vi "INIT.vi"(8 "error in (no error)":errorcluster, 11 "Emulate in":refnum<class "Emulate.lvclass">) -> (0 "error out":errorcluster, 3 "Emulate out":refnum<class "Emulate.lvclass">)   [LabVIEW 2020, in "Emulate.lvclass"]
uses:
  Emulate.lvclass
  C:/Dev/TRANCON/Classes/GeneralFunctionality/GeneralFunctionality.lvclass
  C:/Dev/TRANCON/Classes/Detector/Detector.lvclass
  GeneralFunctionality/GeneralFunctionality.lvclass/GeneralFunctionality.ctl
  Config/Config.lvclass
  Detector.lvclass
  Emulate.lvclass/Emulate.ctl
  GeneralFunctionality/GeneralFunctionality.lvclass
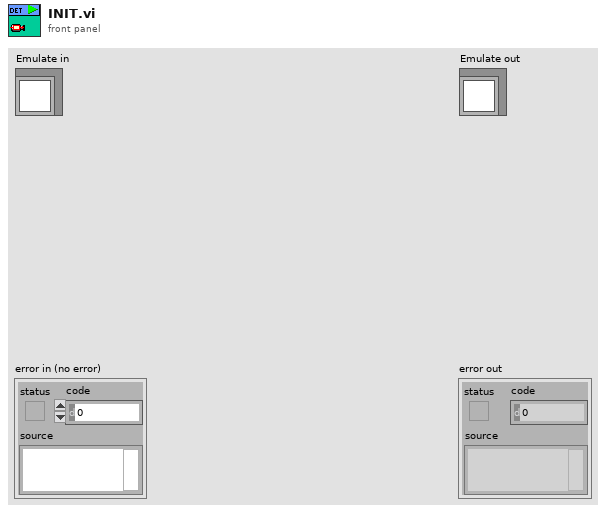
[diagram p1: front panel]
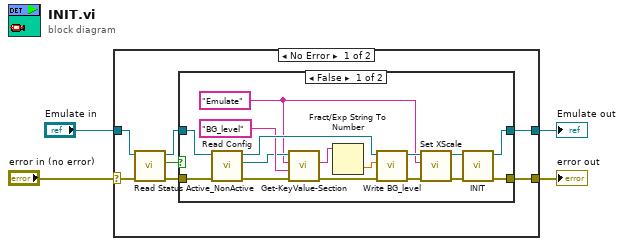
[diagram p0: block diagram]
diagram:
  n1 = case shown="No Error" "error in (no error)" {
    selector: "error in (no error)" -> [w11 w30]
    tunnel: "Emulate in" -> [w10 w31]
    tunnel: [w8 w31] -> w2
    tunnel: [w6 w30] -> w1
    frame No Error {
      n2 = call "Read Status Active_NonActive.vi"("error in (no error)"=w11, "GeneralFunctionality in"=w10) -> ("error out"=w5:errorcluster, "Status Active/NonActive"=w9:bool, "GeneralFunctionality out"=w7:refnum<class "Emulate.lvclass">)  [unwired: 7 in]
      n3 = case shown="False" w9 {
        tunnel: [w13 w29] -> w8
        tunnel: w7 -> [w18 w29]
        tunnel: [w12 w28] -> w6
        tunnel: w5 -> [w17 w28]
        frame False {
          w16 = "Emulate" ("Section")
          n4 = call "Read Config.vi"("error in (no error)"=w17, "GeneralFunctionality en entrée"=w18) -> ("error out"=w19:errorcluster, "Config.lvclass"=w20:refnum<class "Config.lvclass">, "GeneralFunctionality en sortie"=w25:refnum<class "Emulate.lvclass">)  [unwired: 7 in]
          n5 = call-dynamic "Get-KeyValue-Section.vi"("error in (no error)"=w19, "Key"="BG_level", "Section"=w16, "Config in"=w20) -> ("error out"=w21:errorcluster, "Value"=w23:string)  [unwired: 5 in, 1 out]
          n6 = Fract/Exp String To Number(string=w23) -> (number=w24:dbl)  [unwired: 3 in, 1 out]
          n7 = call-dynamic "Write BG_level.vi"("error in (no error)"=w21, "BG_level"=w24, "Detector in"=w25) -> ("error out"=w27:errorcluster, "Detector out"=w26:refnum<class "Emulate.lvclass">)  [unwired: 7 in]
          n8 = call "Set XScale.vi"("error in (no error)"=w27, "Section"=w16, "Detector en entrée"=w26) -> ("error out"=w15:errorcluster, "Detector en sortie"=w14:refnum<class "Emulate.lvclass">)  [unwired: 7 in]
          n9 = call-parent "INIT.vi"("error in (no error)"=w15, "Detector in"=w14) -> ("error out"=w12:errorcluster, "Detector out"=w13:refnum<class "Emulate.lvclass">)  [unwired: 8 in]
        }
        frame True {
        }
      }
    }
    frame Error {
    }
  }
  "error out" <- w1
  "Emulate out" <- w2
